vi "Send Configure Standard Waveform [STD].vi"(2 "dc offset (0.00 V)":dbl[unit] format="%.3f", 4 "amplitude (1.00 V)":dbl[unit]=1.0 format="%.3f", 5 "start phase (0.00 Degrees)":dbl[unit] format="%.3f", 6 "frequency (1000.0 Hz)":dbl[unit]=1000.0 format="%^.2e", 7 "Message Priority (Normal)":T1=enum."Normal", 8 "error in (no error)":errorcluster, 9 "waveform (Sine)":i32(ring)=1 items=["Sine"=1, "Square"=2, "Triangle"=3, "Ramp Up"=4, "Ramp Down"=5, "DC"=6], 10 "channel name (\"CHANNEL1\")":string="CHANNEL1", 11 "Message Enqueuer":refnum<class "Message Enqueuer.lvclass">) -> (0 "error out":errorcluster, 3 "Message Enqueuer out":refnum<class "Message Enqueuer.lvclass">)   [LabVIEW 2015, in "CS++Fgen.lvlib" / "Configure Standard Waveform [STD] Msg.lvclass"]
doc: "Sends the <B>CS++Fgen.lvlib:Configure Standard Waveform [STD] Msg.lvclass</B> message.\n\n<B>CS++Fgen.lvlib:CS++Fgen.lvclass:Configure Standard Waveform [STD].vi</B> Description:\n\nThis VI configures the properties of the function generator that affect standard waveform generation. These properties are the waveform, amplitude, DC offset, frequency, and start phase.\n\nNotes:\n\n(1) This VI is part of the IviFgenStdFunc [STD] extension group."
uses:
  Configure Standard Waveform [STD] Msg.lvclass
  <vilib>/ActorFramework/Message Enqueuer/Message Enqueuer.lvclass
  <vilib>/ActorFramework/Message Enqueuer/Message Priority.ctl
  Configure Standard Waveform [STD] Msg.lvclass/Configure Standard Waveform [STD] Msg.ctl
  <vilib>/ActorFramework/Message Enqueuer/Message Enqueuer.lvclass/Message Enqueuer.ctl
  <vilib>/ActorFramework/Message Priority Queue/Priority Enqueue.vi
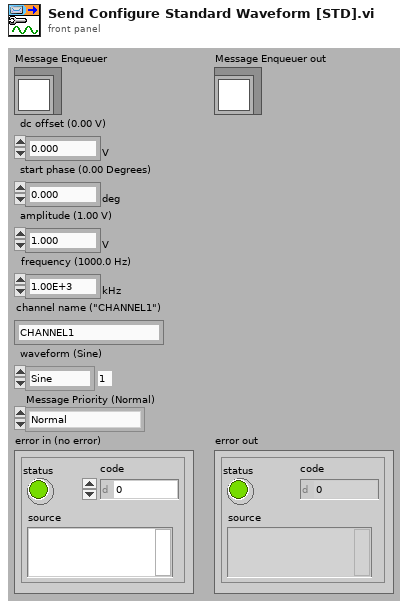
[diagram p1: front panel]
types:
  T1 = typedef "Actor Framework.lvlib/Message Enqueuer.lvclass/Message Priority.ctl" = enum16{"Low", "Normal", "High"}
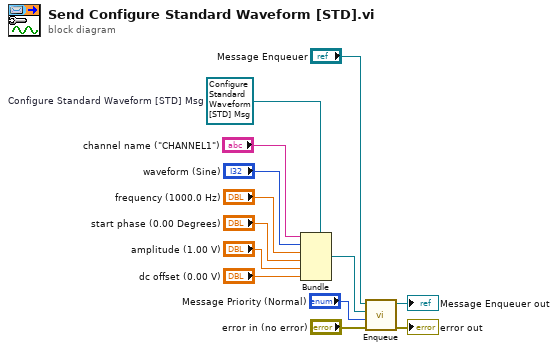
[diagram p0: block diagram]
diagram:
  w7 = refnum<class "Configure Standard Waveform [STD] Msg.lvclass"> refnum  # Configure Standard Waveform [STD] Msg
  n1 = Bundle(cluster=w7, "channel name (\"CHANNEL1\")", "waveform (Sine)", "frequency (1000.0 Hz)", "start phase (0.00 Degrees)", "amplitude (1.00 V)", "dc offset (0.00 V)") -> (w10:refnum<class "Configure Standard Waveform [STD] Msg.lvclass">)
  n2 = call <vilib>:"Enqueue.vi"("error in (no error)"="error in (no error)", "Message Priority (Normal)"="Message Priority (Normal)", "Message"=w10, "Message Enqueuer in"="Message Enqueuer") -> ("error out"=→"error out":errorcluster, "Message Enqueuer out"=→"Message Enqueuer out":refnum<class "Message Enqueuer.lvclass">)  [unwired: 6 in]
